vi "GetStr.vi"(8 "error in (no error)":errorcluster, 11 "reference in":refnum<class "GOOP4_Sub.lvclass">) -> (0 "error out":errorcluster, 2 "Str":string, 3 "reference in":refnum<class "GOOP4_Sub.lvclass">)   [LabVIEW 2020, in "GOOP4_Sub.lvclass"]
uses:
  GOOP4_Sub.lvclass
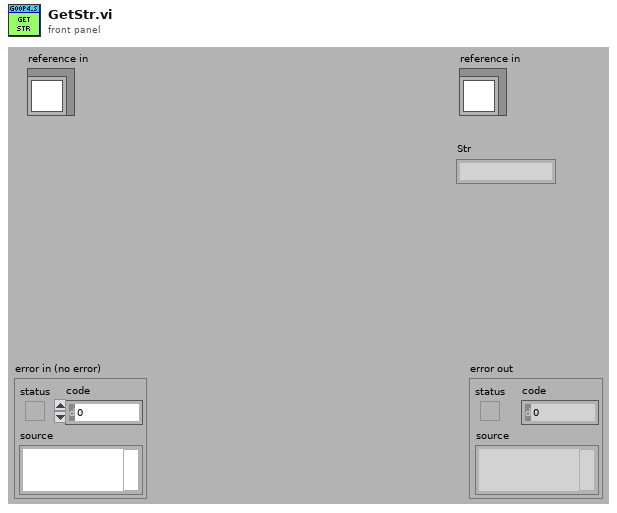
[diagram p1: front panel]
types:
  T1 = typedef "GOOP4_Sub.lvclass/ObjectAttributes.ctl" = cluster{"Str":string}
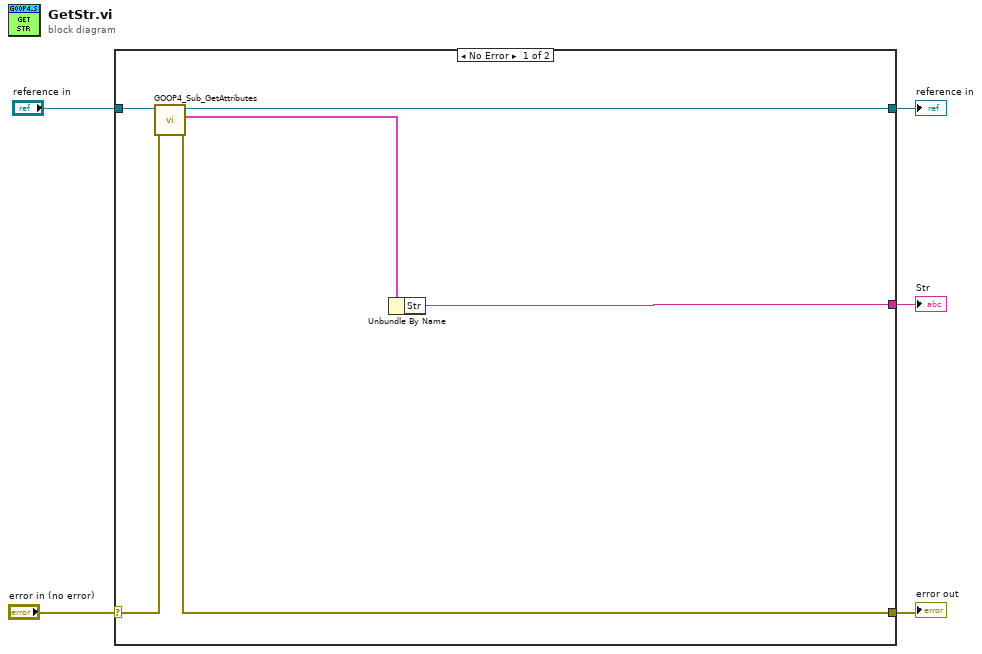
[diagram p0: block diagram]
diagram:
  n1 = case shown="No Error" "error in (no error)" {
    selector: "error in (no error)" -> [w11 w13]
    tunnel: [w9 w13] -> w4
    tunnel: [w7 w12] -> w2
    tunnel: "reference in" -> [w8 w12]
    tunnel: [w6 _] -> w1
    frame No Error {
      n2 = call "GOOP4_Sub_GetAttributes.vi"("error in (no error)"=w11, "reference in"=w8) -> ("error out"=w9:errorcluster, "Data"=w10:T1, "reference out"=w7:refnum<class "GOOP4_Sub.lvclass">)  [unwired: 6 in, 1 out]
      n3 = Unbundle By Name(w10) -> ("Str"=w6:string)
    }
    frame Error {
    }
  }
  "error out" <- w4
  "reference in" <- w2
  "Str" <- w1
